vi "Query USB Connection Status.vi"(8 "error in (no error)":errorcluster, 11 "MC switch refnum in":refnum<k24>) -> (0 "error out":errorcluster, 2 "USB connection active?":bool, 3 "MC switch refnum out":refnum<k24>)   [LabVIEW 2019, in "Minicircuit RF Switch Box.lvlib"]
doc: "Returns the internal temperature (in degrees Celsius) measured at 1 of the internal sensors (model dependent):\n\n- USB-1SPDT-A18 / RC-1SPDT-A18 (1 sensor)\n- USB-1SP4T-A18 / RC-1SP4T-A18 (1 sensor)\n- RC-2MTS-18 (2 sensors)\n- USB-2SPDT-A18 / RC-2SPDT-A18 (2 sensors)\n- USB-3SPDT-A18 / RC-3SPDT-A18 (2 sensors)\n- USB-4SPDT-A18 / RC-4SPDT-A18 (2 sensors)\n- USB-8SPDT-A18 / RC-8SPDT-A18 (3 sensors)\n- RC-2SP4T-x (2 sensors)\n- RC-2SP6T-A12 (2 sensors)\n\nNote: Units with serial numbers earlier than 11108010000 may have a different number of\nsensors than indicated above.\n\nIf a sensor that does not exist is polled (for example there is no sensor 2 on USB-1SPDT-A18)\nthe temperature returned will be “+25.00”"
uses:
  <instrlib>/Minicircuit RF Switch Box/Minicircuit RF Switch Box.lvlib
  C:/Program Files (x86)/National Instruments/LabVIEW 2019/instr.lib/Minicircuit RF Switch Box/mcl_RF_Switch_Controller_NET45.dll
  mcl_RF_Switch_Controller_NET45.dll
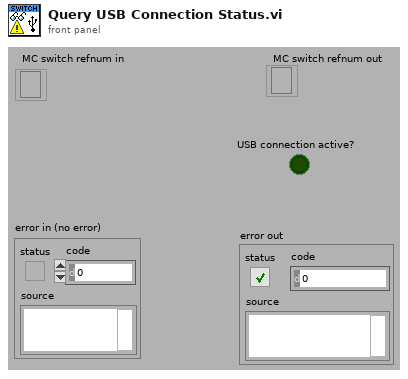
[diagram p1: front panel]
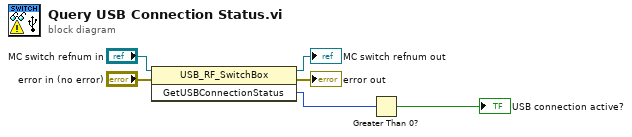
[diagram p0: block diagram]
diagram:
  n1 = invoke class="USB_RF_SwitchBox" method="GetUSBConnectionStatus"(reference="MC switch refnum in", error in="error in (no error)") -> (reference out=→"MC switch refnum out":refnum<k24>, error out=→"error out":errorcluster, "GetUSBConnectionStatus"=w2:i32)  [unwired: 1 in]
  n2 = Greater Than 0?(x=w2) -> (x > 0?=→"USB connection active?":bool)
